vi "BotSpeak.Com.vi"(1 "To Send":string, 2 "Bot Settings in":T1) -> (3 "error out":errorcluster, 4 "Sent":string, 5 "Reply":string, 6 "Bot Settings out":T1)   [LabVIEW 2014]
uses:
  <userlib>/botspeakLib/VIs/Direct/BotSpeak_Control.ctl
  <userlib>/botspeakLib/VIs/SubVIs/BotSpeak_Globals.vi
panel:
  out "Numeric":i32
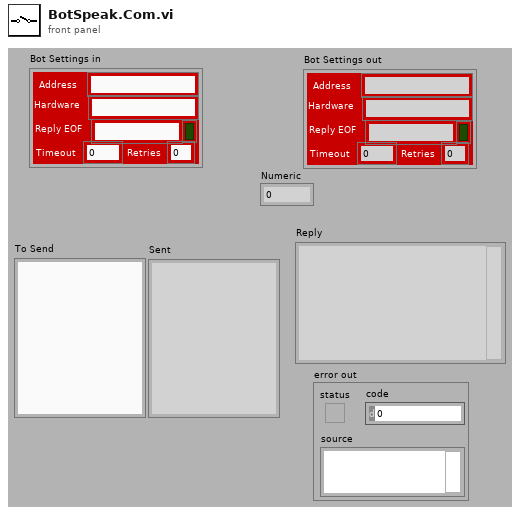
[diagram p1: front panel]
types:
  T1 = typedef "BotSpeak_Control.ctl" = cluster{"Address":string, "Reply EOF":string, "Hardware":string, "Retries":i8, "Timeout":i32, "Open?":bool}
  T2 = typedef "BotSpeak.HardwareSpecs.ctl" = cluster{"Hardware Name":string, "Hardware URL":string, "ComType":enum16{"Undefined", "HTTP", "Serial", "TCPIP", "Console"}, "TCP Port":i32, "DefaultAddress":string, "Retries":i32, "Translate":enum16{"None", "Tiny", "URAPI"}, "MaxScriptSize":i32, "MaxVarNumber":i32, "StartupWait":i32, "Patience":i32, "Startup Patience":i32, "Hardware Help":string, "Com Protocol":string, "Translator":cluster{"BotSpeak CMD":string, "CMD out":string}[], "Init Code":string, "Variable Format":enum16{"INT", "FLOAT", "FIXED"}, "username":string, "password":string}
  T3 = cluster{"BotSpeak CMD":string, "CMD out":string}[]
  T4 = enum16{"Undefined", "HTTP", "Serial", "TCPIP", "Console"}
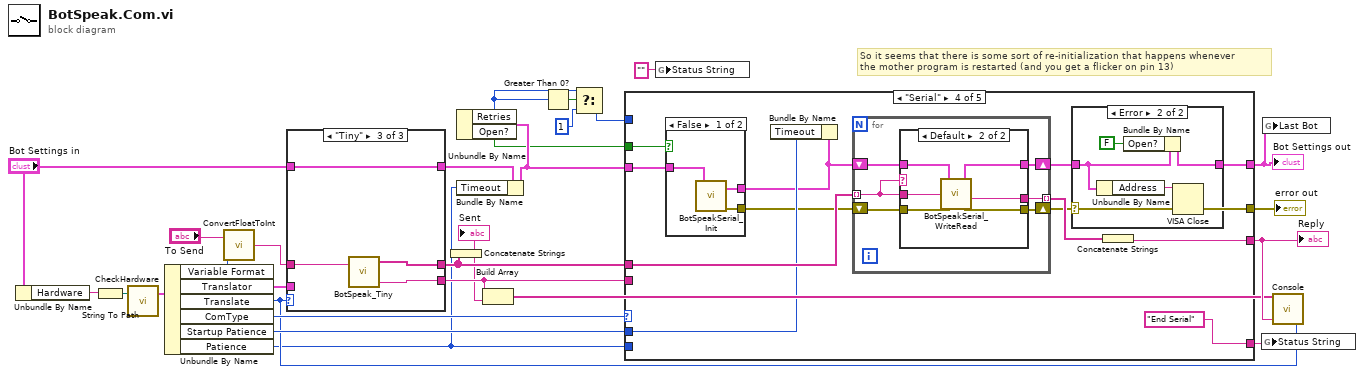
[diagram p0: block diagram]
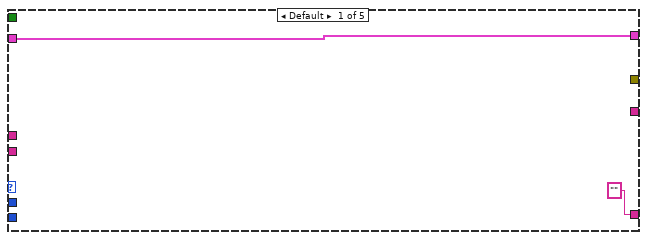
[diagram p2: hidden frame]
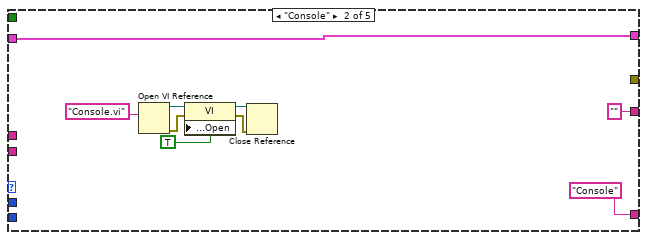
[diagram p3: hidden frame]
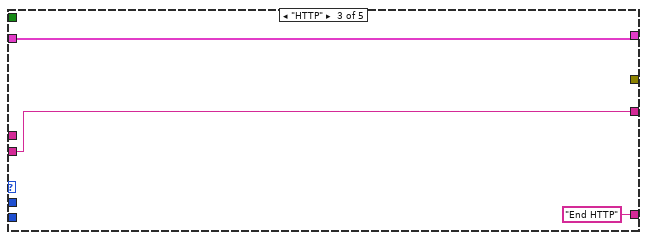
[diagram p4: hidden frame]
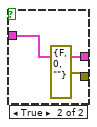
[diagram p6: hidden frame]
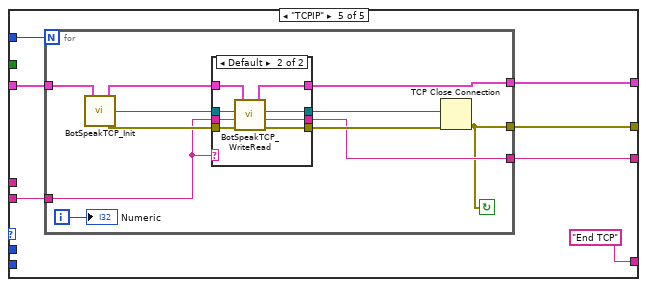
[diagram p8: hidden frame]
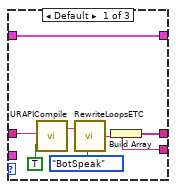
[diagram p10: hidden frame]
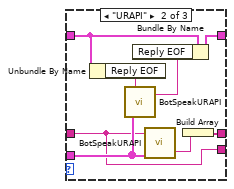
[diagram p11: hidden frame]
diagram:
  # "So it seems that there is some sort of re-initialization that happens whenever\nthe mother program is restarted (and you get a flicker on pin 13)"
  n1 = Unbundle By Name("Bot Settings in") -> ("Hardware"=w27:string)
  n2 = String To Path(string=w27) -> (path=w10:path)
  n3 = call <userlib>:"CheckHardware.vi"("Hardware"=w10) -> ("HardwareSpecs"=w23:T2)  [unwired: 2 in]
  n4 = Unbundle By Name(w23) -> ("Variable Format"=w11:enum16{"INT", "FLOAT", "FIXED"}, "Translator"=w22:T3, "Translate"=w14:enum16{"None", "Tiny", "URAPI"}, "ComType"=w26:T4, "Startup Patience"=w21:i32, "Patience"=w8:i32)
  n5 = call <userlib>:"ConvertFloatToInt.vi"("Variable Format"=w11, "To Send in"="To Send") -> ("To Send out"=w12:string)
  n6 = case shown="\"Tiny\"" w14 {
    tunnel: w12 -> [w30 w36 w47]
    tunnel: [w34 w37 w46] -> w28
    tunnel: w22 -> [_ w42 _]
    tunnel: [w35 w40 w45] -> w9
    tunnel: "Bot Settings in" -> [w35 w41 w45]
    tunnel: [w31 w36 w44] -> w18
    frame Default {
      n7 = call <userlib>:"URAPICompile.vi"("Comments?"=TRUE, "Script"=w30) -> ("trimmed script"=w32:string)
      n8 = call <userlib>:"RewriteLoopsETC.vi"("Type"=enum16{"Tiny", "BotSpeak"}."BotSpeak", "URAPI in"=w32) -> ("URAPI out"=w31:string)
      n9 = Build Array(w31) -> (w34:string[])
    }
    frame "URAPI" {
      n10 = Unbundle By Name(w41) -> ("Reply EOF"=w43:string)
      n11 = call <userlib>:"BotSpeakURAPI.vi"("Translator"=w42, "To Send"=w43) -> ("translated"=w39:string)  [unwired: 1 out]
      n12 = Bundle By Name(cluster=w41, "Reply EOF"=w39) -> (w40:T1)
      n13 = call <userlib>:"BotSpeakURAPI.vi"("Translator"=w42, "To Send"=w36) -> ("translated w \\n"=w38:string)  [unwired: 1 out]
      n14 = Build Array(w38) -> (w37:string[])
    }
    frame "Tiny" {
      n15 = call <userlib>:"BotSpeak_Tiny.vi"("URAPI"=w47) -> ("URAPI  2"=w44:string, "Tiny Lines"=w46:string[])  [unwired: 1 in, 1 out]
    }
  }
  n16 = Concatenate Strings(w28) -> (w17:string)
  "Sent" <- w17
  n17 = Bundle By Name(cluster=w9, "Timeout"=w8) -> (w6:T1)
  n18 = Unbundle By Name(w6) -> ("Retries"=w3:i8, "Open?"=w5:bool)
  n19 = Build Array(w18, w17) -> (w15:string[])
  n20 = Greater Than 0?(x=w3) -> (x > 0?=w4:bool)
  n21 = Select(t=w3, s=w4, f=i8 1) -> (s? t:f=w1:i8)
  n22 = case shown="\"Serial\"" w26 {
    tunnel: w28 -> [_ _ _ w73 _]
    tunnel: [_ "" ("data out") w60 w68 w101] -> w16
    tunnel: [_ _ _ w62 w103] -> w25
    tunnel: w6 -> [w49 w58 w61 w72 w104]
    tunnel: [w49 w58 w61 w65 w105] -> w7
    tunnel: w21 -> [_ _ _ w71 _]
    tunnel: ["" ("Status String") "Console" ("Status String") "End HTTP" ("Status String") "End Serial" ("Status String") "End TCP" ("Status String")] -> w20
    tunnel: w18 -> [_ _ w60 _ w100]
    tunnel: w8 -> [_ _ _ _ _]
    tunnel: w5 -> [_ _ _ w64 _]
    tunnel: w1 -> [_ _ _ _ w99]
    frame Default {
    }
    frame "Console" {
      n23 = Open VI Reference(vi path="Console.vi" ("Status String")) -> (vi reference=w55:refnum<vi>, error out=w54:errorcluster)  [unwired: 5 in]
      n24 = property class="VI"(reference=w55, error in=w54, "Front Panel.Open"=TRUE ("Front Panel Window:Open")) -> (reference out=w51:refnum<vi>, error out=w52:errorcluster)
      n25 = Close Reference(reference=w51, error in (no error)=w52) -> ()  [unwired: 1 out]
    }
    frame "HTTP" {
    }
    frame "Serial" {
      n26 = case shown="False" w64 {
        tunnel: w72 -> [w81 w83]
        tunnel: [w80 w83] -> w63
        tunnel: [w79 errorcluster {"status"=FALSE, "code"=0, "source"=""} ("error out")] -> w66
        frame False {
          n27 = call <userlib>:"BotSpeakSerial_Init.vi"("Bot Settings in"=w81) -> ("error out"=w79:errorcluster, "Bot Settings out"=w80:T1)  [unwired: 1 in]
        }
        frame True {
        }
      }
      n28 = Bundle By Name(cluster=w63, "Timeout"=w71) -> ()  [unwired: 1 out]
      n29 = for {
        tunnel: w73 -> [w84] mode=indexing
        tunnel: [w89] -> w69 mode=indexing
        shift-right: [w85] -> w67
        shift-left: w63 -> [w88]
        shift-right: [w86] -> w62
        shift-left: w66 -> [w87]
        n30 = case shown="Default" w84 {
          tunnel: w84 -> [w90 w98]
          tunnel: [w90 w97] -> w89
          tunnel: w88 -> [w92 w96]
          tunnel: w87 -> [w91 w95]
          tunnel: [w91 w94] -> w86
          tunnel: [w92 w93] -> w85
          frame "" {
          }
          frame Default {
            n31 = call <userlib>:"BotSpeakSerial_WriteRead.vi"("error In"=w95, "To Write"=w98, "Bot Settings in"=w96) -> ("error out"=w94:errorcluster, "Reply"=w97:string, "Bot Settings out"=w93:T1)  [unwired: 1 out]
          }
        }
      }
      n32 = case shown="Error" w62 {
        tunnel: w67 -> [w74 w78]
        tunnel: [w74 w77] -> w65
        frame No Error {
        }
        frame Error {
          n33 = Unbundle By Name(w78) -> ("Address"=w76:string)
          n34 = Bundle By Name(cluster=w78, "Open?"=FALSE) -> (w77:T1)
          n35 = VISA Close(VISA resource name=w76) -> ()  [unwired: 1 in, 1 out]
        }
      }
      n36 = Concatenate Strings(w69) -> (w68:string)
    }
    frame "TCPIP" {
      n37 = for {
        N: w99 -> [_]
        tunnel: [w115] -> w105
        tunnel: w104 -> [w112]
        tunnel: [w107] -> w103
        tunnel: [w109] -> w101
        tunnel: w100 -> [w108]
        i -> [w106]
        stop <- w107 continue-if-true
        n38 = call <userlib>:"BotSpeakTCP_Init.vi"("Bot Settings in"=w112) -> ("error out"=w113:errorcluster, "connection ID"=w114:refnum<k5>, "Bot Settings out"=w116:T1)  [unwired: 1 in]
        n39 = case shown="Default" w108 {
          tunnel: w116 -> [w120 w128]
          tunnel: [w120 w127] -> w115
          tunnel: w114 -> [w119 w126]
          tunnel: w113 -> [w117 w125]
          tunnel: [w119 w124] -> w111
          tunnel: [w117 w123] -> w110
          tunnel: [w118 w122] -> w109
          tunnel: w108 -> [w118 w121]
          frame "" {
          }
          frame Default {
            n40 = call <userlib>:"BotSpeakTCP_WriteRead.vi"("error in"=w125, "To Send"=w121, "connection ID"=w126, "Bot Settings in"=w128) -> ("error out"=w123:errorcluster, "data out"=w122:string, "connection ID out"=w124:refnum<k5>, "Bot Settings out"=w127:T1)
          }
        }
        n41 = TCP Close Connection(connection ID=w111, error in (no error)=w110) -> (error out=w107:errorcluster)  [unwired: 1 in, 1 out]
        "Numeric" <- w106
      }
    }
  }
  "Reply" <- w16
  "error out" <- w25
  "Bot Settings out" <- w7
  n42 = global write "BotSpeak_Globals.vi" "Status String"("" ("Status String")) -> ()
  n43 = global write "BotSpeak_Globals.vi" "Status String"(w20) -> ()
  n44 = global write "BotSpeak_Globals.vi" "Last Bot"(w7) -> ()
  n45 = call <userlib>:"Console.vi"("Translate"=w14, "Reply"=w16, "Sent"=w15) -> ()  [unwired: 1 in, 2 out]
